vi "CSMKVMap-Read.vi"(5 "name":string, 6 "Error in":errorcluster caption="Error in (no error)", 9 "default value (empty variant)":variant) -> (0 "Error out":errorcluster, 3 "value":variant)   [LabVIEW 2017, in "Communicable State Machine.lvlib"]
uses:
  Communicable State Machine.lvlib
  ChangeFlag/ChangeFlag-Read.vi
  ChangeFlag/ChangeFlag-Write.vi
  Utility/Random Change Flag.vi
  ChangeFlag/ChangeFlagDB.vi
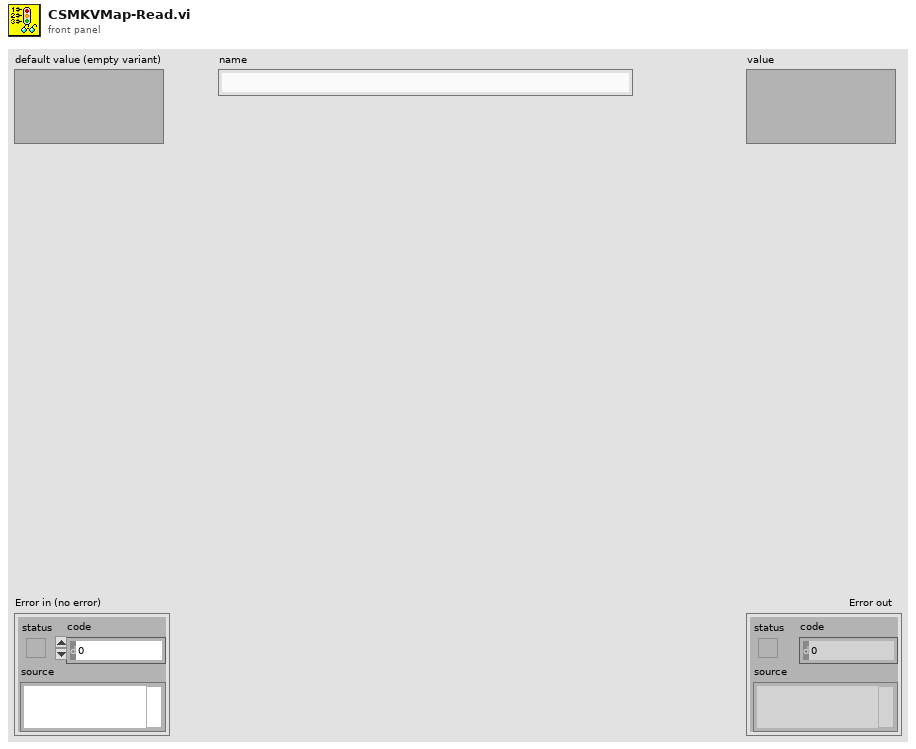
[diagram p1: front panel]
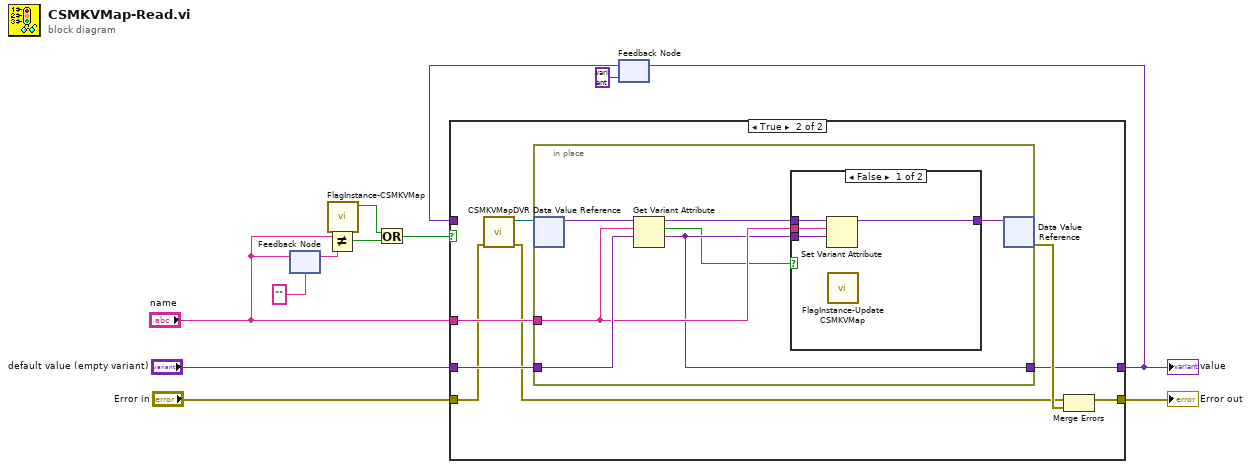
[diagram p0: block diagram]
diagram:
  n1 = feedback #1("" ("name")) -> (w9:string)
  n2 = feedback-in #1("name") -> ()
  n3 = Not Equal?(x="name", y=w9) -> (x != y?=w6:bool)
  n4 = call "FlagInstance-CSMKVMap.vi"() -> ("Changed"=w5:bool)  [unwired: 10 in, 1 out]
  n5 = Or(x=w5, y=w6) -> (x .or. y?=w4:bool)
  n6 = feedback #2(variant ("default value (empty variant)")) -> (w2:variant)
  n7 = case shown="True" w4 {
    tunnel: "name" -> [_ w22]
    tunnel: "Error in" -> [w14 w16]
    tunnel: [w14 w21] -> w11
    tunnel: "default value (empty variant)" -> [_ w19]
    tunnel: [w13 w18] -> w3
    tunnel: w2 -> [w13 _]
    frame False {
    }
    frame True {
      n8 = call "CSMKVMapDVR.vi"("error in (no error)"=w16) -> ("error out"=w15:errorcluster, "KVMapDVR"=w17:refnum<data-value>)  [unwired: 9 in]
      n9 = in-place {
        in-place-border: w22 -> [w25]
        in-place-border: w19 -> [w27]
        in-place-border: [w24] -> w18
        n10 = in-place-dvr #3(w17) -> (w29:variant)  [unwired: 1 out]
        n11 = Get Variant Attribute(Variant=w29, name=w25, default value (empty Variant)=w27) -> (duplicate Variant=w28:variant, found=w23:bool, value=w24:variant)  [unwired: 1 in, 1 out]
        n12 = case shown="False" w23 {
          tunnel: w28 -> [w33 w34]
          tunnel: [w32 w34] -> w26
          tunnel: w25 -> [w31 _]
          tunnel: w24 -> [w30 _]
          frame False {
            n13 = Set Variant Attribute(Variant=w33, name=w31, value=w30) -> (Variant out=w32:variant)  [unwired: 1 in, 2 out]
            n14 = call "FlagInstance-Update CSMKVMap.vi"() -> ()  [unwired: 10 in, 2 out]
          }
          frame True {
          }
        }
        n15 = in-place-dvr #3(w26) -> (w20:errorcluster)  [unwired: 1 out]
      }
      n16 = Merge Errors(w15, w20) -> (w21:errorcluster)
    }
  }
  "Error out" <- w11
  "value" <- w3
  n17 = feedback-in #2(w3) -> ()
